vi "AH read data.vi"(8 "error in (no error)":errorcluster, 11 "VISA Resource Name":refnum<visa-resource-name>) -> (0 "error out":errorcluster, 1 "Loss":dbl, 2 "Capacitance":dbl, 3 "VISA Resource Name Out":refnum<visa-resource-name>)   [LabVIEW 2019]
panel:
  out "x-y 3":u32
  out "x-y 2":u32
  out "x-y":u32
  out "Numeric":i32
  in  "address":i16
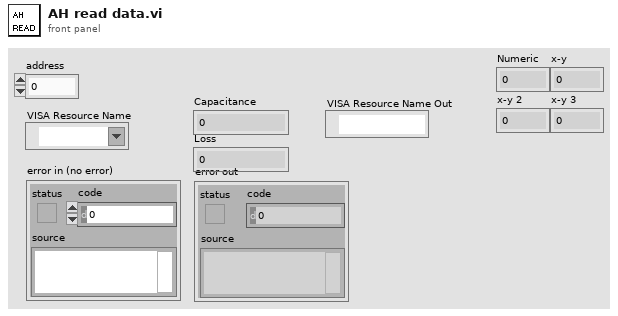
[diagram p1: front panel]
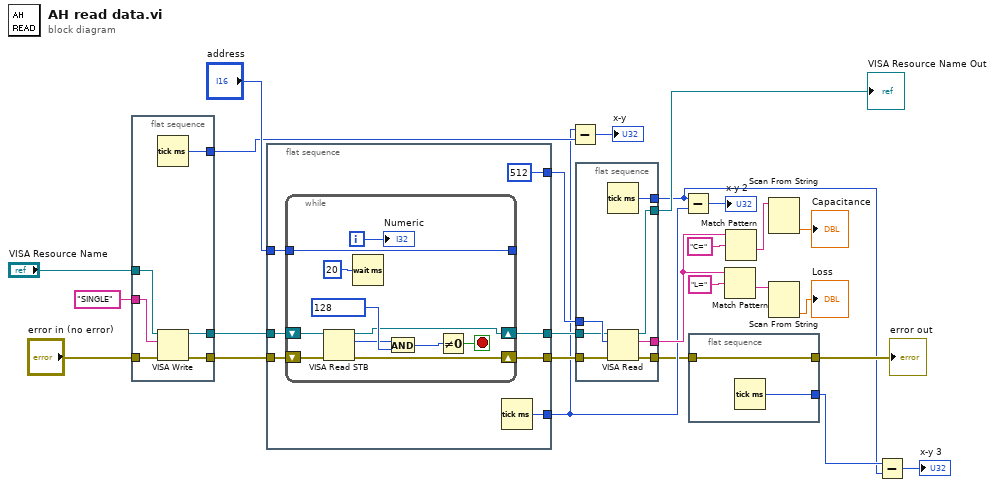
[diagram p0: block diagram]
diagram:
  n1 = flat-sequence {
    tunnel: [w32] -> w20
    tunnel: "error in (no error)" -> [w31]
    tunnel: "SINGLE" ("write buffer") -> [w30]
    tunnel: "VISA Resource Name" -> [w29]
    tunnel: [w28] -> w13
    tunnel: [w27] -> w9
    frame #0 {
      n2 = Tick Count (ms)() -> (millisecond timer value=w27:u32)
      n3 = VISA Write(VISA resource name=w29, write buffer=w30, error in (no error)=w31) -> (VISA resource name out=w28:refnum<visa-resource-name>, error out=w32:errorcluster)  [unwired: 1 out]
    }
  }
  n4 = flat-sequence {
    tunnel: w20 -> [w39]
    tunnel: "address" -> [w38]
    tunnel: [w37] -> w17
    tunnel: [u32 512 ("read count")] -> w16
    tunnel: w13 -> [w35]
    tunnel: [w34] -> w12
    tunnel: [w33] -> w8
    frame #0 {
      n5 = while {
        tunnel: w38 -> [w44]
        shift-right: [w45] -> w37
        shift-left: w39 -> [w50]
        tunnel: [w44] -> _
        shift-right: [w42] -> w34
        shift-left: w35 -> [w43]
        i -> [w40]
        stop <- w47 stop-if-true
        n6 = VISA Read STB(8:w50, 11:w43) -> (0:w45:errorcluster, 2:w41:u16, 3:w42:refnum<visa-resource-name>)
        n7 = Wait (ms)(milliseconds to wait=u32 20) -> ()  [unwired: 1 out]
        n8 = And(x=w41, y=u16 128) -> (x .and. y?=w48:u16)
        n9 = Not Equal To 0?(x=w48) -> (x != 0?=w47:bool)
        "Numeric" <- w40
      }
      n10 = Tick Count (ms)() -> (millisecond timer value=w33:u32)
    }
  }
  n11 = Subtract(x=w8, y=w9) -> (x-y=→"x-y":u32)
  n12 = flat-sequence {
    tunnel: [w57] -> w7
    tunnel: w17 -> [w56]
    tunnel: w16 -> [w55]
    tunnel: w12 -> [w54]
    tunnel: [w53] -> w11
    tunnel: [w52] -> w10
    tunnel: [w51] -> w4
    frame #0 {
      n13 = Tick Count (ms)() -> (millisecond timer value=w51:u32)
      n14 = VISA Read(VISA resource name=w54, byte count=w55, error in (no error)=w56) -> (VISA resource name out=w52:refnum<visa-resource-name>, read buffer=w53:string, error out=w57:errorcluster)  [unwired: 1 out]
    }
  }
  n15 = Subtract(x=w4, y=w8) -> (x-y=→"x-y 2":u32)
  n16 = flat-sequence {
    tunnel: w7 -> [w59]
    tunnel: [w59] -> w6
    tunnel: [w58] -> w5
    frame #0 {
      n17 = Tick Count (ms)() -> (millisecond timer value=w58:u32)
    }
  }
  n18 = Match Pattern(string=w11, regular expression="L=") -> (after substring=w22:string)  [unwired: 4 out]
  n19 = Match Pattern(string=w11, regular expression="C=") -> (after substring=w25:string)  [unwired: 4 out]
  n20 = Scan From String(input string=w25) -> (output 1=→"Capacitance":dbl)  [unwired: 3 in, 4 out]
  n21 = Scan From String(input string=w22) -> (output 1=→"Loss":dbl)  [unwired: 3 in, 4 out]
  n22 = Subtract(x=w5, y=w4) -> (x-y=→"x-y 3":u32)
  "error out" <- w6
  "VISA Resource Name Out" <- w10
